vi "LibXML_GetTextChildValue.vi"(4 "error in":errorcluster, 6 "node":u32) -> (0 "error out":errorcluster, 3 "lvstring":string)   [LabVIEW 2019, in "Tools.lvlib" / "LibXML.lvlib"]
uses:
  LibXML.lvlib
  LibXML_NavigateDirection.ctl
  LibXML_GetNodeStrPtr.vi
  LibXML_GetNodeResolvedContentStrPointer.vi
  LibXML_GetStringLength.vi
  LibXML_CopyString.vi
  Error Cluster From Error Code_subroutine.vi
  <vilib>/Utility/error.llb/Trim Whitespace.vi
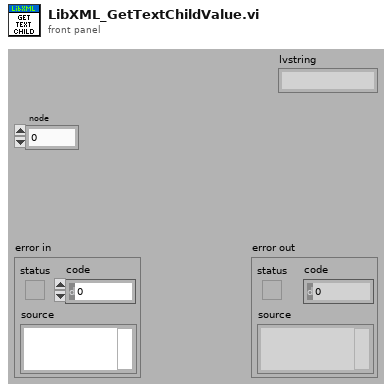
[diagram p1: front panel]
types:
  T1 = enum16{"nothing", "element", "attribute", "text", "cdata", "5 or more"}
  T2 = typedef "Tools.lvlib/LibXML.lvlib/LibXML_NavigateDirection.ctl" = enum16{"NOP", "first child", "last child", "parent", "next", "prev"}
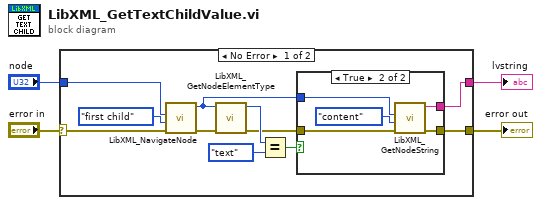
[diagram p0: block diagram]
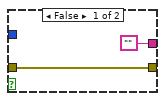
[diagram p2: hidden frame]
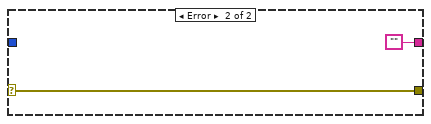
[diagram p3: hidden frame]
diagram:
  n1 = case shown="No Error" "error in" {
    selector: "error in" -> [w15 w24]
    tunnel: [w8 w24] -> w3
    tunnel: "node" -> [w6 _]
    tunnel: [w5 ""] -> w1
    frame No Error {
      n2 = call "LibXML_NavigateNode.vi"("error in (no error)"=w15, "direction"=LibXML_NavigateDirection."first child", "node in"=w6) -> ("error out"=w13:errorcluster, "node out"=w9:u32)  [unwired: 2 in, 1 out]
      n3 = call "LibXML_GetNodeElementType.vi"("error in"=w13, "node"=w9) -> ("error out"=w10:errorcluster, "element type"=w12:T1)  [unwired: 7 in, 1 out]
      n4 = Equal?(x=w12, y=T1."text") -> (x = y?=w7:bool)
      n5 = case shown="True" w7 {
        tunnel: w10 -> [w16 w22]
        tunnel: w9 -> [_ w20]
        tunnel: [w16 w19] -> w8
        tunnel: ["" ("lvstring") w18] -> w5
        frame False {
        }
        frame True {
          n6 = call "LibXML_GetNodeString.vi"("error in"=w22, "type"=enum16{"NOP", "name", "content"}."content", "node"=w20) -> ("error out"=w19:errorcluster, "lvstring"=w18:string)  [unwired: 7 in]
        }
      }
    }
    frame Error {
    }
  }
  "error out" <- w3
  "lvstring" <- w1
